vi "3.2.vi"(1 "B":dbl, 2 "功能选择":enum16{"相除", "相乘", "相减", "相加"}(ring), 3 "A":dbl) -> (0 "结果":dbl)   [LabVIEW 2017]
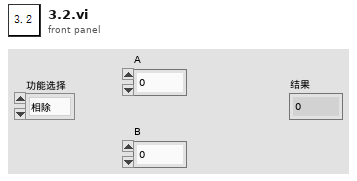
[diagram p1: front panel]
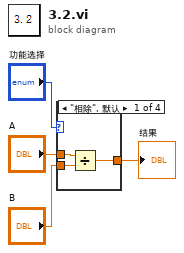
[diagram p0: block diagram]
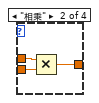
[diagram p2: hidden frame]
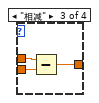
[diagram p3: hidden frame]
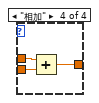
[diagram p4: hidden frame]
diagram:
  n1 = case shown="\"相除\", 默认" "功能选择" {
    tunnel: "A" -> [w7 w10 w13 w16]
    tunnel: "B" -> [w6 w9 w12 w15]
    tunnel: [w5 w8 w11 w14] -> w1
    frame "相除", Default {
      n2 = Divide(x=w7, y=w6) -> (x/y=w5:dbl)
    }
    frame "相乘" {
      n3 = Multiply(x=w10, y=w9) -> (x*y=w8:dbl)
    }
    frame "相减" {
      n4 = Subtract(x=w13, y=w12) -> (x-y=w11:dbl)
    }
    frame "相加" {
      n5 = Add(x=w16, y=w15) -> (x+y=w14:dbl)
    }
  }
  "结果" <- w1
